vi "mod_Interpolating FIR (re+im).vi"(0 "Real in":dbl[](array[numeric]), 1 "Reset":bool, 5 "Im in":dbl[](array[numeric]), 9 "interpolation":i32, 11 "error in (no error)":errorcluster, 12 "taps":dbl[](array[numeric])) -> (4 "Real out":dbl[](array[numeric]), 6 "im out":dbl[](array[numeric]), 15 "error out":errorcluster)   [LabVIEW 2020, in "niAMT.lvlib"]
uses:
  <vilib>/addons/Modulation/niAMT.lvlib
  <vilib>/Analysis/3filter.llb/IIR Filter with I.C..vi
  <vilib>/Analysis/3filter.llb/IIR Filter with I.C. (DBL).vi
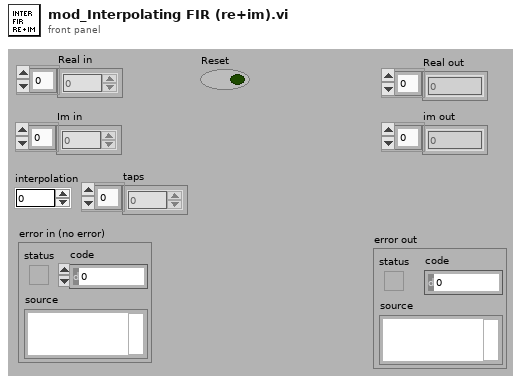
[diagram p1: front panel]
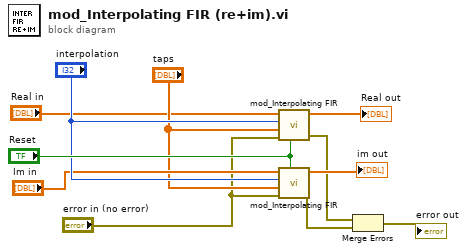
[diagram p0: block diagram]
diagram:
  n1 = call <vilib>:"mod_Interpolating FIR.vi"("reset"="Reset", "error in (no error)"="error in (no error)", "taps"="taps", "interpolation"="interpolation", "x"="Real in") -> ("error out"=w3:errorcluster, "filtered x"=→"Real out":dbl[])  [unwired: 3 out]
  n2 = call <vilib>:"mod_Interpolating FIR.vi"("reset"="Reset", "error in (no error)"="error in (no error)", "taps"="taps", "interpolation"="interpolation", "x"="Im in") -> ("error out"=w2:errorcluster, "filtered x"=→"im out":dbl[])  [unwired: 3 out]
  n3 = Merge Errors(w3, w2) -> (→"error out":errorcluster)
